vi "Actor Core.vi"(8 "error in":errorcluster, 11 "CameraTestingUI in":refnum<class "CameraTestingENI.lvclass">) -> (0 "error out":errorcluster, 3 "Actor out":refnum<class "Actor.lvclass">)   [LabVIEW 2020, in "CameraTestingProxy.lvlib" / "CameraTestingENI.lvclass"]
doc: "(<B>Filename</B>: Actor Framework.lvlib:Actor.lvclass:Actor Core.vi)\n\nReceives messages to the actor, reacts to them, and initiates any error handling that may shut the actor down.\n\nDescendant classes may override this VI to append parallel tasks for the actor to complete while it handles messages. Overrides use the Call Parent Class Method node."
uses:
  CameraTestingENI.lvclass
  <vilib>/ActorFramework/Actor/Actor.lvclass
  <vilib>/ActorFramework/Message Enqueuer/Message Enqueuer.lvclass
  CameraTestingENI.lvclass/CameraTestingENI.ctl
  Private/TypeDef/HelperLoopCamTestEvn.ctl
  Camera/ICamera/ICamera/TypeDef/SnapInfo.ctl
  CameraTestingApp/ICameraTesting/ICameraTesting/TypeDef/FrameRateValReceived.ctl
  CameraTestingApp/ICameraTesting/ICameraTesting/TypeDef/ImgTypeValReceived.ctl
  CameraTestingApp/ICameraTesting/ICameraTesting/TypeDef/ResolutionValReceived.ctl
  CameraTestingApp/ICameraTesting/ICameraTesting/TypeDef/VideoOptCodesUpdated.ctl
  CameraTestingApp/ICameraTesting/ICameraTesting/TypeDef/VideoOptionsInfo.ctl
  CameraTestingApp/ICameraTesting/ICameraTesting/TypeDef/StatusUpdated.ctl
  CameraTestingApp/ICameraTesting/ICameraTesting/TypeDef/StatusRecord.ctl
  ICameraTestingProxy/ICameraTestingProxy/TypeDef/SnapData.ctl
  ICameraTestingProxy/ICameraTestingProxy/TypeDef/Resolution.ctl
  <vilib>/ActorFramework/Message Enqueuer/Message Enqueuer.lvclass/Message Enqueuer.ctl
  CameraTestingApp/ICameraTesting/ICameraTesting Messages/SetFrameRate Msg/SetFrameRate Msg.lvclass/SetFrameRate Msg.ctl
  CameraTestingApp/ICameraTesting/ICameraTesting Messages/SetImageType Msg/SetImageType Msg.lvclass/SetImageType Msg.ctl
  CameraTestingApp/ICameraTesting/ICameraTesting Messages/SetResolution Msg/SetResolution Msg.lvclass/SetResolution Msg.ctl
  Private/TypeDef/VideoLoopCamTestEvn.ctl
  CameraTestingApp/ICameraTesting/ICameraTesting/TypeDef/VideoBufferUpdate.ctl
  ICameraTestingProxy/ICameraTestingProxy/TypeDef/VideoFrameData.ctl
  f73fc735-489c-4749-bae7-300f2c0ce07b.vi
  3a7c0926-b8ef-4989-a529-ecf0d899ca9b.vi
  f7a01f60-f3aa-429c-834c-31ca40de0e93.vi
  7ad3a5b3-60c8-426a-bbf4-9e0d3f24ac53.vi
  2cc18511-968a-477e-8b3d-f91ca7a54db9.vi
  76229903-142a-4204-acbb-6e81851a6772.vi
  d734633a-91e4-4fcd-8cf9-d7cd2009acdc.vi
  1f239cb3-5779-402d-b8a0-3f2b57b93c48.vi
  45aa87c6-b464-47c1-b1de-58be862de037.vi
  <vilib>/ActorFramework/Message Enqueuer/Enqueue.vi
  CameraTestingApp/ICameraTesting/ICameraTesting Messages/DisconnectCamera Msg/DisconnectCamera Msg.lvclass
  C:/Program Files (x86)/National Instruments/LabVIEW 2020/vi.lib/ActorFramework/Message/Message.lvclass
  CameraTestingApp/ICameraTesting/ICameraTesting Messages/ConnectCamera Msg/ConnectCamera Msg.lvclass
  CameraTestingApp/ICameraTesting/ICameraTesting Messages/GetFrameRate Msg/GetFrameRate Msg.lvclass
  CameraTestingApp/ICameraTesting/ICameraTesting Messages/GetImageType Msg/GetImageType Msg.lvclass
  CameraTestingApp/ICameraTesting/ICameraTesting Messages/GetResolution Msg/GetResolution Msg.lvclass
  CameraTestingApp/ICameraTesting/ICameraTesting Messages/SetFrameRate Msg/SetFrameRate Msg.lvclass
  CameraTestingApp/ICameraTesting/ICameraTesting Messages/SetImageType Msg/SetImageType Msg.lvclass
  CameraTestingApp/ICameraTesting/ICameraTesting Messages/SetResolution Msg/SetResolution Msg.lvclass
  CameraTestingApp/ICameraTesting/ICameraTesting Messages/StopStreaming Msg/StopPlayMsg.lvclass
  CameraTestingApp/ICameraTesting/ICameraTesting Messages/StartStreaming Msg/StartPlay Msg.lvclass
  CameraTestingApp/ICameraTesting/ICameraTesting Messages/SingleShot Msg/SingleShot Msg.lvclass
  CameraTestingApp/ICameraTesting/ICameraTesting Messages/AcqVideoOptCodes Msg/AcqVideoOptCodes Msg.lvclass
  <vilib>/ActorFramework/Stop Msg/Stop Msg.lvclass
  <vilib>/ActorFramework/Message Priority Queue/Priority Enqueue.vi
  CameraTestingApp/ICameraTesting/ICameraTesting/ICameraTesting.lvclass
  ICameraTestingProxy/ICameraTestingProxy/ICameraTestingProxy.lvclass
  Camera/ICamera/ICamera/ICamera.lvclass
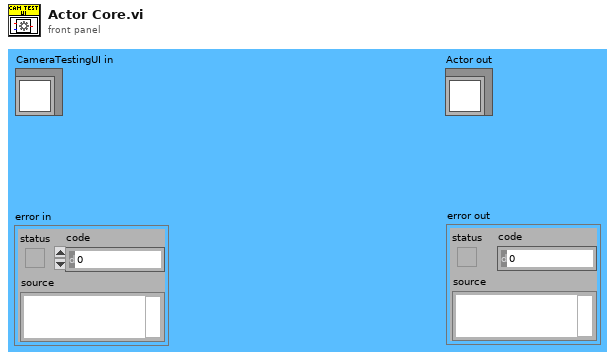
[diagram p1: front panel]
types:
  T1 = typedef "CameraTestingProxy.lvlib/CameraTestingENI.lvclass/HelperLoopEvntRegRef.ctl" = refnum<event-registration>
  T2 = typedef "CameraTestingProxy.lvlib/CameraTestingENI.lvclass/VideoLoopEnvRgstRef.ctl" = refnum<event-registration>
  T3 = typedef "CameraTestingProxy.lvlib/CameraTestingENI.lvclass/HelperLoopCamTestEvn.ctl" = cluster{"NewSnapData":refnum<user-event>, "FrameRateValReceived":T4, "ImgTypeValReceived":T5, "ResolutionValReceived":T6, "VideoOptInfoUpdated":T7, "StatusUpdated":T8}
  T4 = typedef "ICameraTesting.lvlib/ICameraTesting.lvclass/FrameRateValReceived.ctl" = refnum<user-event>
  T5 = typedef "ICameraTesting.lvlib/ICameraTesting.lvclass/ImgTypeValReceived.ctl" = refnum<user-event>
  T6 = typedef "ICameraTesting.lvlib/ICameraTesting.lvclass/ResolutionValReceived.ctl" = refnum<user-event>
  T7 = typedef "ICameraTesting.lvlib/ICameraTesting.lvclass/VideoOptCodesUpdated.ctl" = refnum<user-event>
  T8 = typedef "ICameraTesting.lvlib/ICameraTesting.lvclass/StatusUpdated.ctl" = refnum<user-event>
  T9 = typedef "ICameraTestingProxy.lvlib/ICameraTestingProxy.lvclass/SnapData.ctl" = cluster{"image depth":i32, "PixelData":u8[], "Resolution":T10}
  T10 = typedef "ICameraTestingProxy.lvlib/ICameraTestingProxy.lvclass/Resolution.ctl" = cluster{"Width":i16, "Height":i16}
  T11 = typedef "ICameraTesting.lvlib/ICameraTesting.lvclass/VideoOptionsInfo.ctl" = cluster{"FrameRateCodesList":cluster{"Description":string, "Code":u8}[], "VideoResolutionCodesList":cluster{"Description":string, "Code":u8}[], "ImageTypeCodesList":cluster{"Description":string, "Code":u8}[]}
  T12 = typedef "CameraTestingProxy.lvlib/CameraTestingENI.lvclass/VideoLoopCamTestEvn.ctl" = cluster{"VideoBufferUpdate":T13}
  T13 = typedef "ICameraTesting.lvlib/ICameraTesting.lvclass/VideoBufferUpdate.ctl" = refnum<user-event>
  T14 = typedef "ICameraTestingProxy.lvlib/ICameraTestingProxy.lvclass/VideoFrameData.ctl" = cluster{"image depth":i32, "Data[]":u8[], "Bounds":cluster{"Height":i16, "Width":i16}}
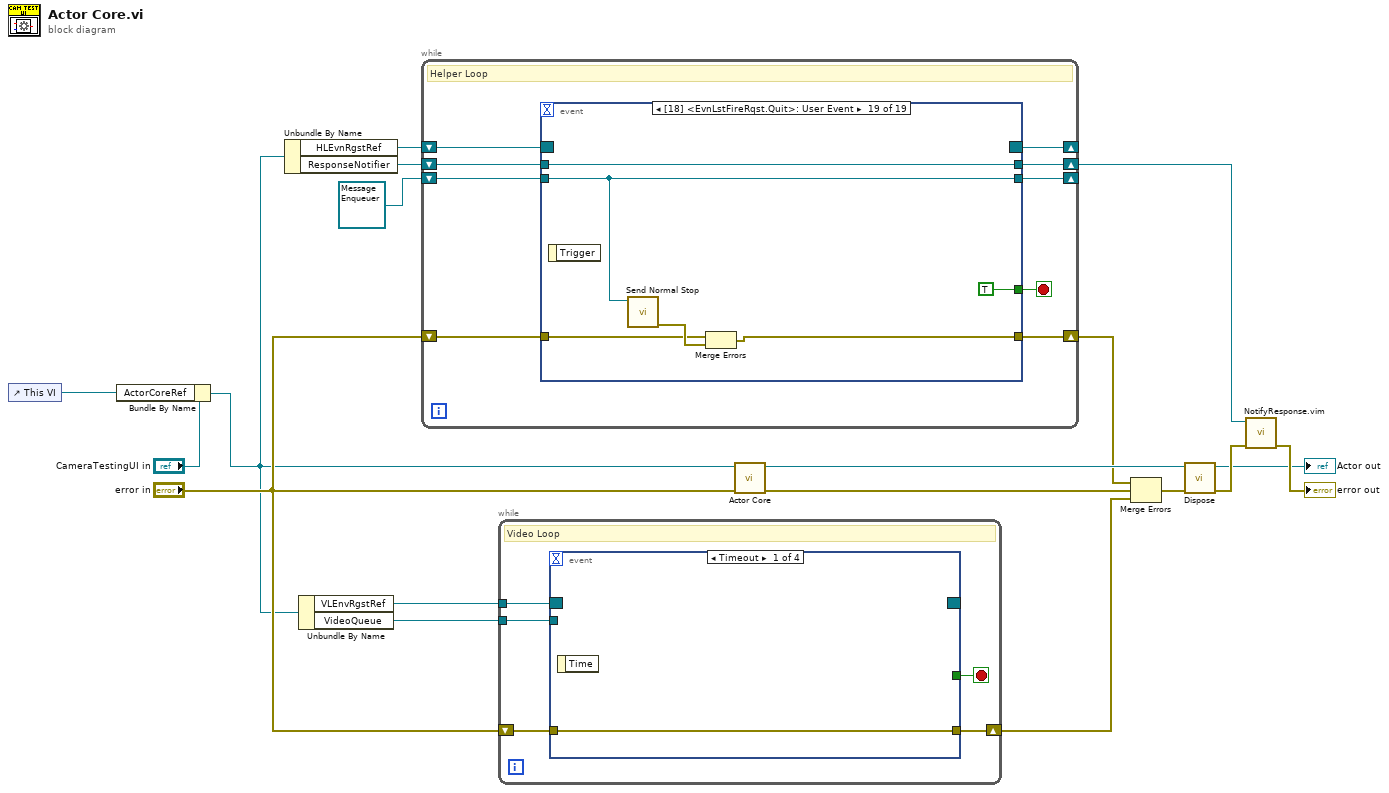
[diagram p0: block diagram]
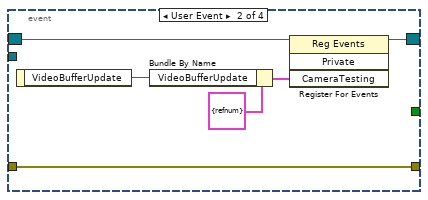
[diagram p2: hidden frame]
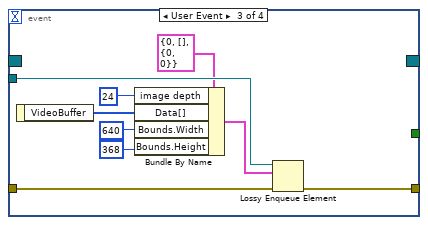
[diagram p3: hidden frame]
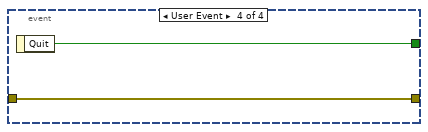
[diagram p4: hidden frame]
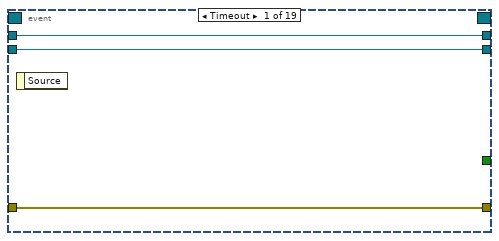
[diagram p5: hidden frame]
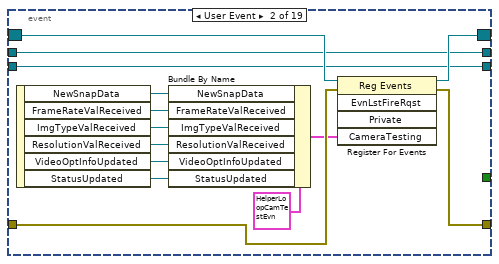
[diagram p6: hidden frame]
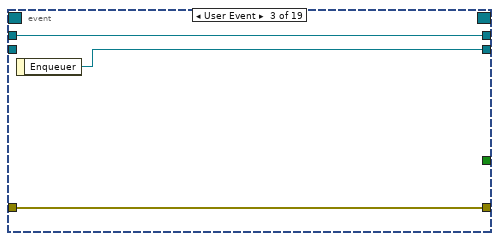
[diagram p7: hidden frame]
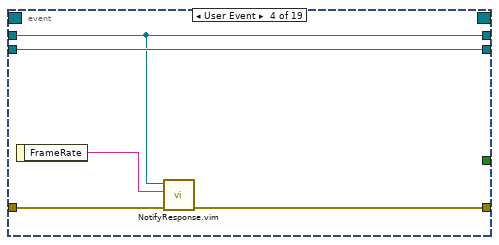
[diagram p8: hidden frame]
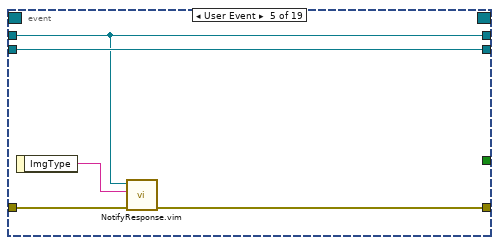
[diagram p9: hidden frame]
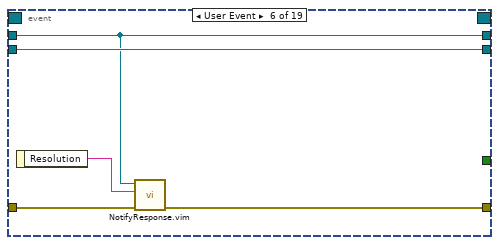
[diagram p10: hidden frame]
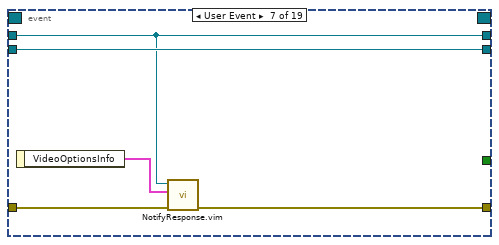
[diagram p11: hidden frame]
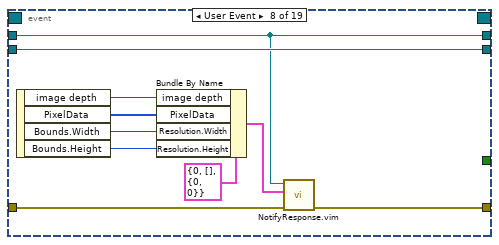
[diagram p12: hidden frame]
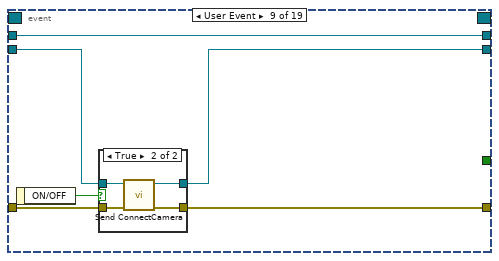
[diagram p13: hidden frame]
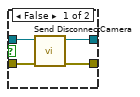
[diagram p14: hidden frame]
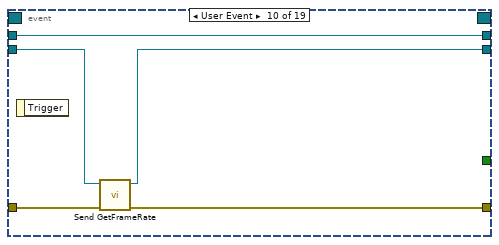
[diagram p15: hidden frame]
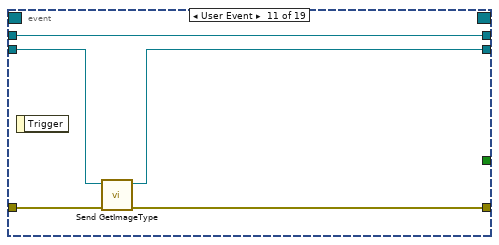
[diagram p16: hidden frame]
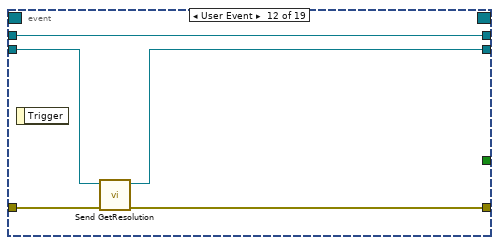
[diagram p17: hidden frame]
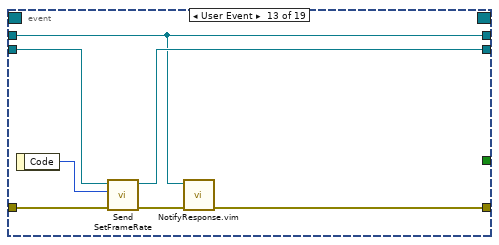
[diagram p18: hidden frame]
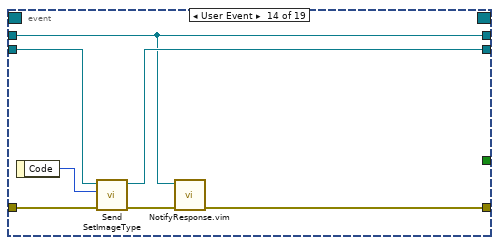
[diagram p19: hidden frame]
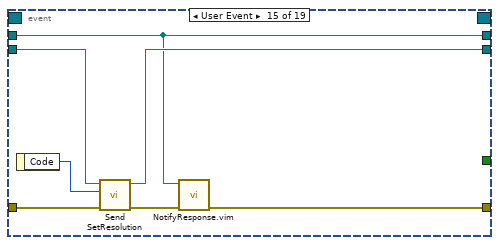
[diagram p20: hidden frame]
diagram:
  n1 = control-ref of="This VI"() -> (w18:refnum<vi>)
  n2 = Bundle By Name(cluster="CameraTestingUI in", "ActorCoreRef"=w18) -> (w5:refnum<class "CameraTestingENI.lvclass">)
  n3 = Unbundle By Name(w5) -> ("HLEvnRgstRef"=w17:T1, "ResponseNotifier"=w8:refnum<notifier>)
  n4 = Unbundle By Name(w5) -> ("VLEnvRgstRef"=w16:T2, "VideoQueue"=w7:refnum<queue>)
  n5 = while {
    shift-right: [w25] -> _
    shift-left: w17 -> [w26]
    shift-right: [w24] -> w11
    shift-left: "error in" -> [w23]
    shift-right: [w22] -> _
    shift-left: refnum<class "Message Enqueuer.lvclass"> refnum ("Message Enqueuer out") -> [w27]
    shift-right: [w20] -> w3
    shift-left: w8 -> [w21]
    stop <- w19 stop-if-true
    # "Helper Loop"
    n6 = event shown="[18] <EvnLstFireRqst.Quit>: User Event" {
      selector: w26 -> [_ w44 _ _ _ _ _ _ _ _ _ _ _ _ _ _ _ _ _]
      dyn-events: [_ w43 _ _ _ _ _ _ _ _ _ _ _ _ _ _ _ _ _] -> w25
      timeout: _ -> [_ _ _ _ _ _ _ _ _ _ _ _ _ _ _ _ _ _ _]
      tunnel: w27 -> [w29 w37 _ w51 w57 w62 w67 w76 w83 w93 w98 w104 w112 w119 w125 w132 w144 w151 w153]
      tunnel: w23 -> [w30 w41 w45 w52 w53 w58 w63 w77 w82 w95 w100 w105 w113 w120 w127 w131 w146 w150 w155]
      tunnel: [w30 w40 w45 w50 w54 w59 w64 w73 w81 w94 w99 w103 w108 w116 w121 w130 w145 w149 w154] -> w24
      tunnel: [w29 w37 w47 w51 w57 w62 w67 w76 w80 w92 w97 w102 w111 w118 w124 w129 w143 w148 w153] -> w22
      tunnel: w21 -> [w28 w38 w46 w49 w55 w60 w66 w72 w78 w96 w101 w106 w107 w115 w123 w128 w142 w147 w157]
      tunnel: [w28 w38 w46 w49 w55 w60 w66 w72 w78 w96 w101 w106 w107 w115 w123 w128 w142 w147 w157] -> w20
      tunnel: [_ _ _ _ _ _ _ _ _ _ _ _ _ _ _ _ _ _ TRUE] -> w19
      event Timeout {
        n7 = event-data() -> ()  [unwired: 1 in, 1 out]
      }
      event User Event {
        n8 = event-data() -> ("NewSnapData"=w36:refnum<user-event>, "FrameRateValReceived"=w35:T4, "ImgTypeValReceived"=w34:T5, "ResolutionValReceived"=w33:T6, "VideoOptInfoUpdated"=w32:T7, "StatusUpdated"=w31:T8)  [unwired: 1 in]
        n9 = Bundle By Name(cluster=T3 {"NewSnapData"=refnum, "FrameRateValReceived"=refnum, "ImgTypeValReceived"=refnum, "ResolutionValReceived"=refnum, "VideoOptInfoUpdated"=refnum, "StatusUpdated"=refnum} ("HelperLoopEvn"), "NewSnapData"=w36, "FrameRateValReceived"=w35, "ImgTypeValReceived"=w34, "ResolutionValReceived"=w33, "VideoOptInfoUpdated"=w32, "StatusUpdated"=w31) -> (w39:T3)
        n10 = register-events(reference=w44, error in=w41, w39) -> (reference out=w43:T1, error out=w40:errorcluster)  [unwired: 2 in]
      }
      event User Event {
        n11 = event-data() -> ("Enqueuer"=w47:refnum<class "Message Enqueuer.lvclass">)  [unwired: 1 in]
      }
      event User Event {
        n12 = event-data() -> ("FrameRate"=w48:string)  [unwired: 1 in]
        n13 = call "NotifyResponse.vim"("error in (no error)"=w52, "Data"=w48, "ResponseNotifier"=w49) -> ("error out"=w50:errorcluster)  [unwired: 8 in]
      }
      event User Event {
        n14 = event-data() -> ("ImgType"=w56:string)  [unwired: 1 in]
        n15 = call "NotifyResponse.vim"("error in (no error)"=w53, "Data"=w56, "ResponseNotifier"=w55) -> ("error out"=w54:errorcluster)  [unwired: 8 in]
      }
      event User Event {
        n16 = event-data() -> ("Resolution"=w61:string)  [unwired: 1 in]
        n17 = call "NotifyResponse.vim"("error in (no error)"=w58, "Data"=w61, "ResponseNotifier"=w60) -> ("error out"=w59:errorcluster)  [unwired: 8 in]
      }
      event User Event {
        n18 = event-data() -> ("VideoOptionsInfo"=w65:T11)  [unwired: 1 in]
        n19 = call "NotifyResponse.vim"("error in (no error)"=w63, "Data"=w65, "ResponseNotifier"=w66) -> ("error out"=w64:errorcluster)  [unwired: 8 in]
      }
      event User Event {
        n20 = event-data() -> ("image depth"=w71:i32, "PixelData"=w70:u8[], "Bounds.Width"=w69:i16, "Bounds.Height"=w68:i16)  [unwired: 1 in]
        n21 = Bundle By Name(cluster=T9 {"image depth"=0, "PixelData"=[], "Resolution"={"Width"=0, "Height"=0}} ("SnapData"), "image depth"=w71, "PixelData"=w70, "Resolution.Width"=w69, "Resolution.Height"=w68) -> (w74:T9)
        n22 = call "NotifyResponse.vim"("error in (no error)"=w77, "Data"=w74, "ResponseNotifier"=w72) -> ("error out"=w73:errorcluster)  [unwired: 8 in]
      }
      event User Event {
        n23 = event-data() -> ("ON/OFF"=w79:bool)  [unwired: 1 in]
        n24 = case shown="True" w79 {
          tunnel: w83 -> [w87 w91]
          tunnel: w82 -> [w85 w90]
          tunnel: [w84 w89] -> w81
          tunnel: [w86 w88] -> w80
          frame False {
            n25 = call "Send DisconnectCamera.vi"("error in (no error)"=w85, "Message Enqueuer"=w87) -> ("error out"=w84:errorcluster, "Message Enqueuer out"=w86:refnum<class "Message Enqueuer.lvclass">)  [unwired: 8 in]
          }
          frame True {
            n26 = call "Send ConnectCamera.vi"("error in (no error)"=w90, "Message Enqueuer"=w91) -> ("error out"=w89:errorcluster, "Message Enqueuer out"=w88:refnum<class "Message Enqueuer.lvclass">)  [unwired: 8 in]
          }
        }
      }
      event User Event {
        n27 = event-data() -> ()  [unwired: 1 in, 1 out]
        n28 = call "Send GetFrameRate.vi"("error in (no error)"=w95, "Message Enqueuer"=w93) -> ("error out"=w94:errorcluster, "Message Enqueuer out"=w92:refnum<class "Message Enqueuer.lvclass">)  [unwired: 8 in]
      }
      event User Event {
        n29 = event-data() -> ()  [unwired: 1 in, 1 out]
        n30 = call "Send GetImageType.vi"("error in (no error)"=w100, "Message Enqueuer"=w98) -> ("error out"=w99:errorcluster, "Message Enqueuer out"=w97:refnum<class "Message Enqueuer.lvclass">)  [unwired: 8 in]
      }
      event User Event {
        n31 = event-data() -> ()  [unwired: 1 in, 1 out]
        n32 = call "Send GetResolution.vi"("error in (no error)"=w105, "Message Enqueuer"=w104) -> ("error out"=w103:errorcluster, "Message Enqueuer out"=w102:refnum<class "Message Enqueuer.lvclass">)  [unwired: 8 in]
      }
      event User Event {
        n33 = event-data() -> ("Code"=w110:u8)  [unwired: 1 in]
        n34 = call "Send SetFrameRate.vi"("error in (no error)"=w113, "Frame Rate"=w110, "Message Enqueuer"=w112) -> ("error out"=w109:errorcluster, "Message Enqueuer out"=w111:refnum<class "Message Enqueuer.lvclass">)  [unwired: 7 in]
        n35 = call "NotifyResponse.vim"("error in (no error)"=w109, "ResponseNotifier"=w107) -> ("error out"=w108:errorcluster)  [unwired: 9 in]
      }
      event User Event {
        n36 = event-data() -> ("Code"=w114:u8)  [unwired: 1 in]
        n37 = call "Send SetImageType.vi"("error in (no error)"=w120, "Image Type"=w114, "Message Enqueuer"=w119) -> ("error out"=w117:errorcluster, "Message Enqueuer out"=w118:refnum<class "Message Enqueuer.lvclass">)  [unwired: 7 in]
        n38 = call "NotifyResponse.vim"("error in (no error)"=w117, "ResponseNotifier"=w115) -> ("error out"=w116:errorcluster)  [unwired: 9 in]
      }
      event User Event {
        n39 = event-data() -> ("Code"=w126:u8)  [unwired: 1 in]
        n40 = call "Send SetResolution.vi"("error in (no error)"=w127, "Resolution"=w126, "Message Enqueuer"=w125) -> ("error out"=w122:errorcluster, "Message Enqueuer out"=w124:refnum<class "Message Enqueuer.lvclass">)  [unwired: 7 in]
        n41 = call "NotifyResponse.vim"("error in (no error)"=w122, "ResponseNotifier"=w123) -> ("error out"=w121:errorcluster)  [unwired: 9 in]
      }
      event User Event {
        n42 = event-data() -> ("ON/OFF"=w133:bool)  [unwired: 1 in]
        n43 = case shown="True" w133 {
          tunnel: w132 -> [w135 w141]
          tunnel: w131 -> [w137 w140]
          tunnel: [w136 w139] -> w130
          tunnel: [w134 w138] -> w129
          frame False {
            n44 = call "Send StopPlay.vi"("error in (no error)"=w137, "Message Enqueuer"=w135) -> ("error out"=w136:errorcluster, "Message Enqueuer out"=w134:refnum<class "Message Enqueuer.lvclass">)  [unwired: 8 in]
          }
          frame True {
            n45 = call "Send StartPlay.vi"("error in (no error)"=w140, "Message Enqueuer"=w141) -> ("error out"=w139:errorcluster, "Message Enqueuer out"=w138:refnum<class "Message Enqueuer.lvclass">)  [unwired: 8 in]
          }
        }
      }
      event User Event {
        n46 = event-data() -> ()  [unwired: 1 in, 1 out]
        n47 = call "Send SingleShot.vi"("error in (no error)"=w146, "Message Enqueuer"=w144) -> ("error out"=w145:errorcluster, "Message Enqueuer out"=w143:refnum<class "Message Enqueuer.lvclass">)  [unwired: 8 in]
      }
      event User Event {
        n48 = event-data() -> ()  [unwired: 1 in, 1 out]
        n49 = call "Send AcqVideoOptCodes.vi"("error in (no error)"=w150, "Message Enqueuer"=w151) -> ("error out"=w149:errorcluster, "Message Enqueuer out"=w148:refnum<class "Message Enqueuer.lvclass">)  [unwired: 8 in]
      }
      event User Event {
        n50 = event-data() -> ()  [unwired: 1 in, 1 out]
        n51 = call <vilib>:"Send Normal Stop.vi"("Message Enqueuer"=w153) -> ("error out"=w156:errorcluster)  [unwired: 10 in]
        n52 = Merge Errors(w155, w156) -> (w154:errorcluster)
      }
    }
  }
  n53 = while {
    tunnel: w16 -> [w162]
    shift-right: [w159] -> w12
    shift-left: "error in" -> [w160]
    tunnel: w7 -> [w158]
    stop <- w161 stop-if-true
    # "Video Loop"
    n54 = event shown="[0] Timeout" {
      selector: w162 -> [_ w169 _ _]
      dyn-events: [_ w168 _ _] -> _
      timeout: _ -> [_ _ _ _]
      tunnel: [_ _ _ w180] -> w161
      tunnel: w160 -> [w163 w164 w178 w179]
      tunnel: [w163 w164 w170 w179] -> w159
      tunnel: w158 -> [_ _ w177 _]
      event Timeout {
        n55 = event-data() -> ()  [unwired: 1 in, 1 out]
      }
      event User Event {
        n56 = event-data() -> ("VideoBufferUpdate"=w167:T13)  [unwired: 1 in]
        n57 = Bundle By Name(cluster=T12 {"VideoBufferUpdate"=refnum} ("event source"), "VideoBufferUpdate"=w167) -> (w165:T12)
        n58 = register-events(reference=w169, w165) -> (reference out=w168:T2)  [unwired: 2 in, 1 out]
      }
      event User Event {
        n59 = event-data() -> ("VideoBuffer"=w172:u8[])  [unwired: 1 in]
        n60 = Bundle By Name(cluster=T14 {"image depth"=0, "Data[]"=[], "Bounds"={"Height"=0, "Width"=0}} ("element"), "image depth"=24, "Data[]"=w172, "Bounds.Width"=i16 640 ("Rectangle.right"), "Bounds.Height"=i16 368 ("Rectangle.bottom")) -> (w171:T14)
        n61 = Lossy Enqueue Element(queue=w177, element=w171, error in (no error)=w178) -> (error out=w170:errorcluster)  [unwired: 3 out]
      }
      event User Event {
        n62 = event-data() -> ("Quit"=w180:bool)  [unwired: 1 in]
      }
    }
  }
  n63 = call-parent "Actor Core.vi"("error in"="error in", "Actor in"=w5) -> ("error out"=w15:errorcluster, "Actor out"=w13:refnum<class "Actor.lvclass">)  [unwired: 8 in]
  n64 = Merge Errors(w11, w15, w12) -> (w14:errorcluster)
  n65 = call "Dispose.vi"("error in (no error)"=w14, "Actor in"=w13) -> ("error out"=w4:errorcluster, "Actor out"=→"Actor out":refnum<class "Actor.lvclass">)  [unwired: 8 in]
  n66 = call "NotifyResponse.vim"("error in (no error)"=w4, "ResponseNotifier"=w3) -> ("error out"=→"error out":errorcluster)  [unwired: 9 in]
